vi "Handle Last Ack Core.vi"(4 "error in (no error)":errorcluster, 6 "Last Ack":refnum<class "Last Ack.lvclass">, 7 "PLC_Module in":refnum<class "PLC_Module.lvclass">) -> (0 "error out":errorcluster, 3 "PLC_Module out":refnum<class "PLC_Module.lvclass">)   [LabVIEW 2025, in "PLC_Module.lvlib" / "PLC_Module.lvclass"]
doc: "<p>(<strong>Filename</strong>: <span class=\"dnl\">Actor Framework.lvlib:Actor.lvclass:Handle Last Ack Core.vi</span>)</p>\n<p>Defines how the caller actor responds to the Last Ack message from a nested actor. The Last Ack message is the final message a nested actor sends to its caller before it shuts down. The message contains information about the final state of the nested actor.</p>\n<p>By default, this method does nothing except return any error the nested actor sent. A descendant class may override this method to define behavior.</p>"
uses:
  PLC_Module.lvclass
  <vilib>/ActorFramework/LastAck/Last Ack.lvclass
  <vilib>/ActorFramework/LastAck/Last Ack.lvclass/Last Ack.ctl
  <vilib>/ActorFramework/Actor/Actor.lvclass
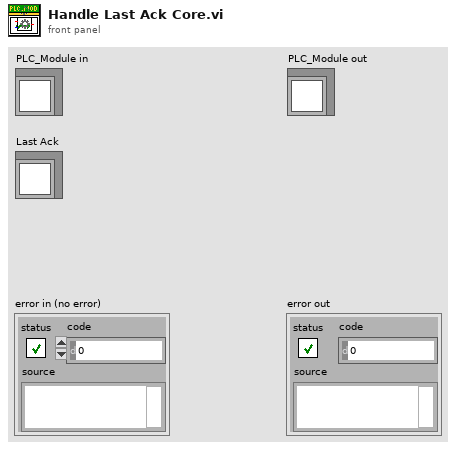
[diagram p1: front panel]
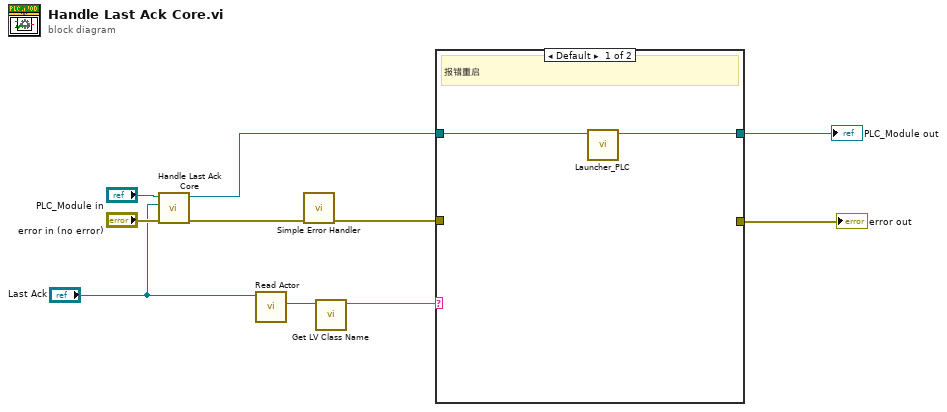
[diagram p0: block diagram]
diagram:
  n1 = call-parent "Handle Last Ack Core.vi"("error in (no error)"="error in (no error)", "Last Ack"="Last Ack", "Actor in"="PLC_Module in") -> ("error out"=w10:errorcluster, "Actor out"=w7:refnum<class "PLC_Module.lvclass">)  [unwired: 3 in]
  n2 = call <vilib>:"Read Actor.vi"("Last Ack"="Last Ack") -> ("Actor"=w2:refnum<class "Actor.lvclass">)  [unwired: 10 in]
  n3 = call <vilib>:"Simple Error Handler.vi"("error in (no error)"=w10) -> ("error out"=w5:errorcluster)  [unwired: 4 in, 4 out]
  n4 = call <vilib>:"Get LV Class Name.vi"("object"=w2) -> ("class name"=w1:string)  [unwired: 9 in, 1 out]
  n5 = case shown="Default" w1 {
    tunnel: w7 -> [w12 w14]
    tunnel: [w11 w14] -> w6
    tunnel: w5 -> [_ w13]
    tunnel: [_ w13] -> w4
    frame Default {
      # "报错重启"
      n6 = call "Launcher_PLC.vi"("PLC_Module in"=w12) -> ("PLC_Module out"=w11:refnum<class "PLC_Module.lvclass">)  [unwired: 9 in, 1 out]
    }
    frame "PLC_Module.lvclass" {
    }
  }
  "PLC_Module out" <- w6
  "error out" <- w4
